vi "Search for Fail.vi"(0 "Results File Path":path, 11 "error in (no error)":errorcluster) -> (4 "String":string, 6 "Pass Status":bool, 15 "error out":errorcluster)   [LabVIEW 2024]
doc: "Searches throught the results file to find failures and format them for display on main FP."
uses:
  <vilib>/Utility/file.llb/Read Delimited Spreadsheet (string).vi
  <userlib>/_OpenG.lib/string/string.llb/openg_string.lvlib
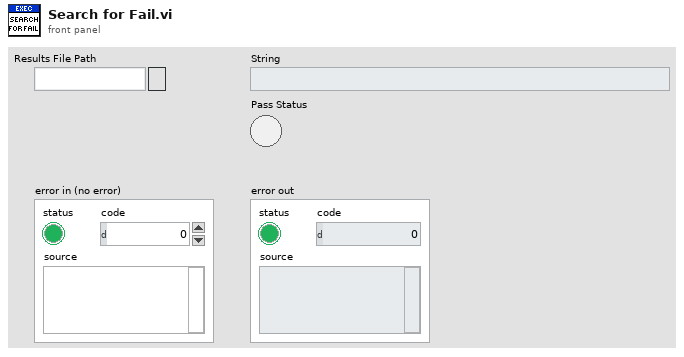
[diagram p1: front panel]
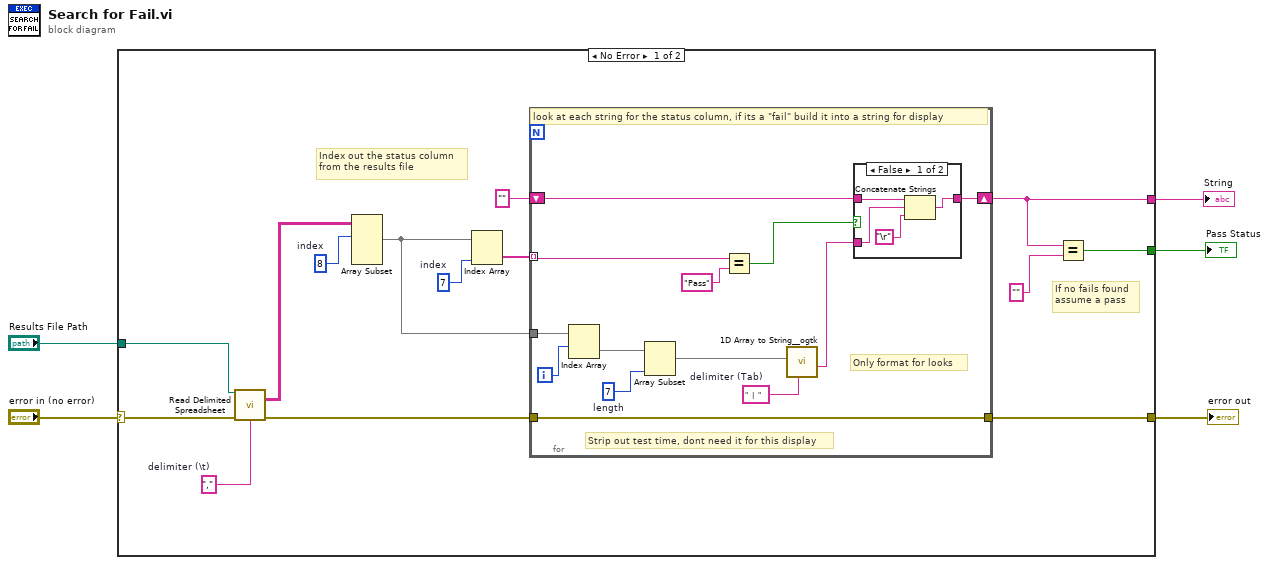
[diagram p0: block diagram]
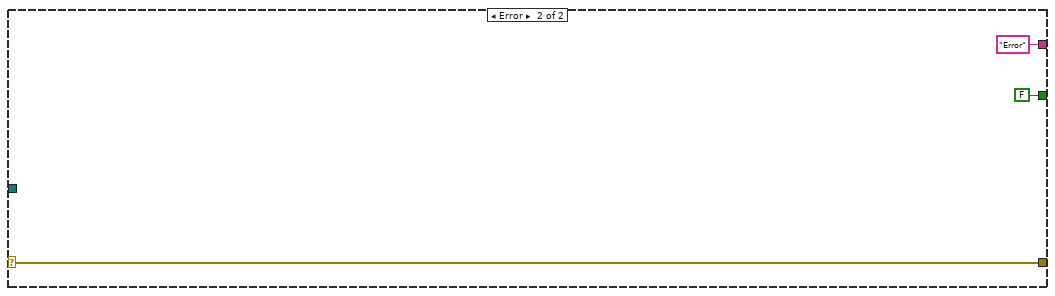
[diagram p3: hidden frame]
diagram:
  n1 = case shown="No Error" "error in (no error)" {
    selector: "error in (no error)" -> [w17 w38]
    tunnel: [w19 w38] -> w5
    tunnel: "Results File Path" -> [w18 _]
    tunnel: [w9 FALSE] -> w2
    tunnel: [w8 "Error"] -> w1
    frame No Error {
      w6 = 7  # index
      w13 = 8  # index
      w10 = ","  # delimiter (\t)
      # "If no fails found\nassume a pass"
      # "Index out the status column\nfrom the results file"
      n2 = call-poly <vilib>:"Read Delimited Spreadsheet.vi"("file path (dialog if empty)"=w18, "error in (no error)"=w17, "delimiter (\\t)"=w10) -> ("all rows"=w11:string[][], "error out"=w16:errorcluster)  [unwired: 7 in, 4 out]
      n3 = Array Subset(array=w11, index (row)=w13) -> (w14:string[][])  [unwired: 3 in]
      n4 = Index Array(array=w14, index (col)=w6) -> (element=w12:string[])  [unwired: 1 in]
      n5 = for {
        tunnel: w12 -> [w32] mode=indexing
        tunnel: w14 -> [w30]
        shift-right: [w26] -> w8
        shift-left: "" -> [w27]
        tunnel: w16 -> [w23]
        tunnel: [w23] -> w19
        i -> [w29]
        w20 = 7  # length
        w24 = "  |  "  # delimiter (Tab)
        # "Only format for looks"
        # "Strip out test time, dont need it for this display"
        # "look at each string for the status column, if its a \"fail\" build it into a string for display"
        n6 = Index Array(array=w30, index (row)=w29) -> (element=w22:string[])  [unwired: 1 in]
        n7 = Array Subset(array=w22, length=w20) -> (w21:string[])  [unwired: 1 in]
        n8 = Equal?(x=w32, y="Pass") -> (x = y?=w28:bool)
        n9 = call <userlib>:"1D Array to String__ogtk.vi"("delimiter (Tab)"=w24, "Array of Strings"=w21) -> ("delimited string"=w25:string)  [unwired: 9 in]
        n10 = case shown="False" w28 {
          tunnel: w25 -> [w35 _]
          tunnel: w27 -> [w36 w37]
          tunnel: [w34 w37] -> w26
          frame False {
            n11 = Concatenate Strings(w36, w35, "\r") -> (w34:string)
          }
          frame True {
          }
        }
      }
      n12 = Equal?(x=w8, y="") -> (x = y?=w9:bool)
    }
    frame Error {
    }
  }
  "String" <- w1
  "error out" <- w5
  "Pass Status" <- w2
